vi "HW 2-2_old.vi"() -> ()   [LabVIEW 2017]
panel:
  in  "MR":bool
  in  "+/-":bool
  out "計算機執行時間":string caption="Elapsed Time Text"
  in  "CE":bool
  in  "1/x":bool
  in  "stop":bool
  out "系統時間":timestamp
  in  ".":bool
  out "String":string
  in  "/":bool
  in  "*":bool
  in  "—":bool
  in  "+":bool
  in  "=":bool
  in  "C":bool
  in  "0":bool
  in  "3":bool
  in  "2":bool
  in  "1":bool
  in  "6":bool
  in  "5":bool
  in  "4":bool
  in  "9":bool
  in  "8":bool
  in  "7":bool
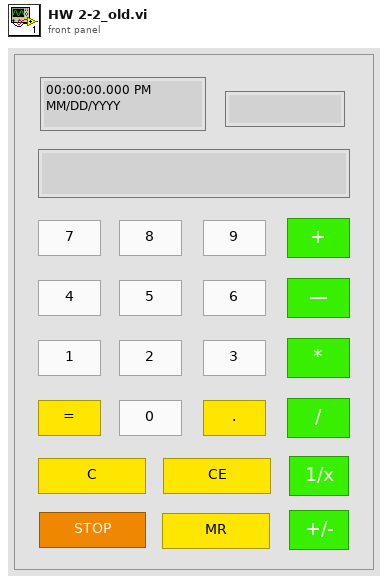
[diagram p1: front panel]
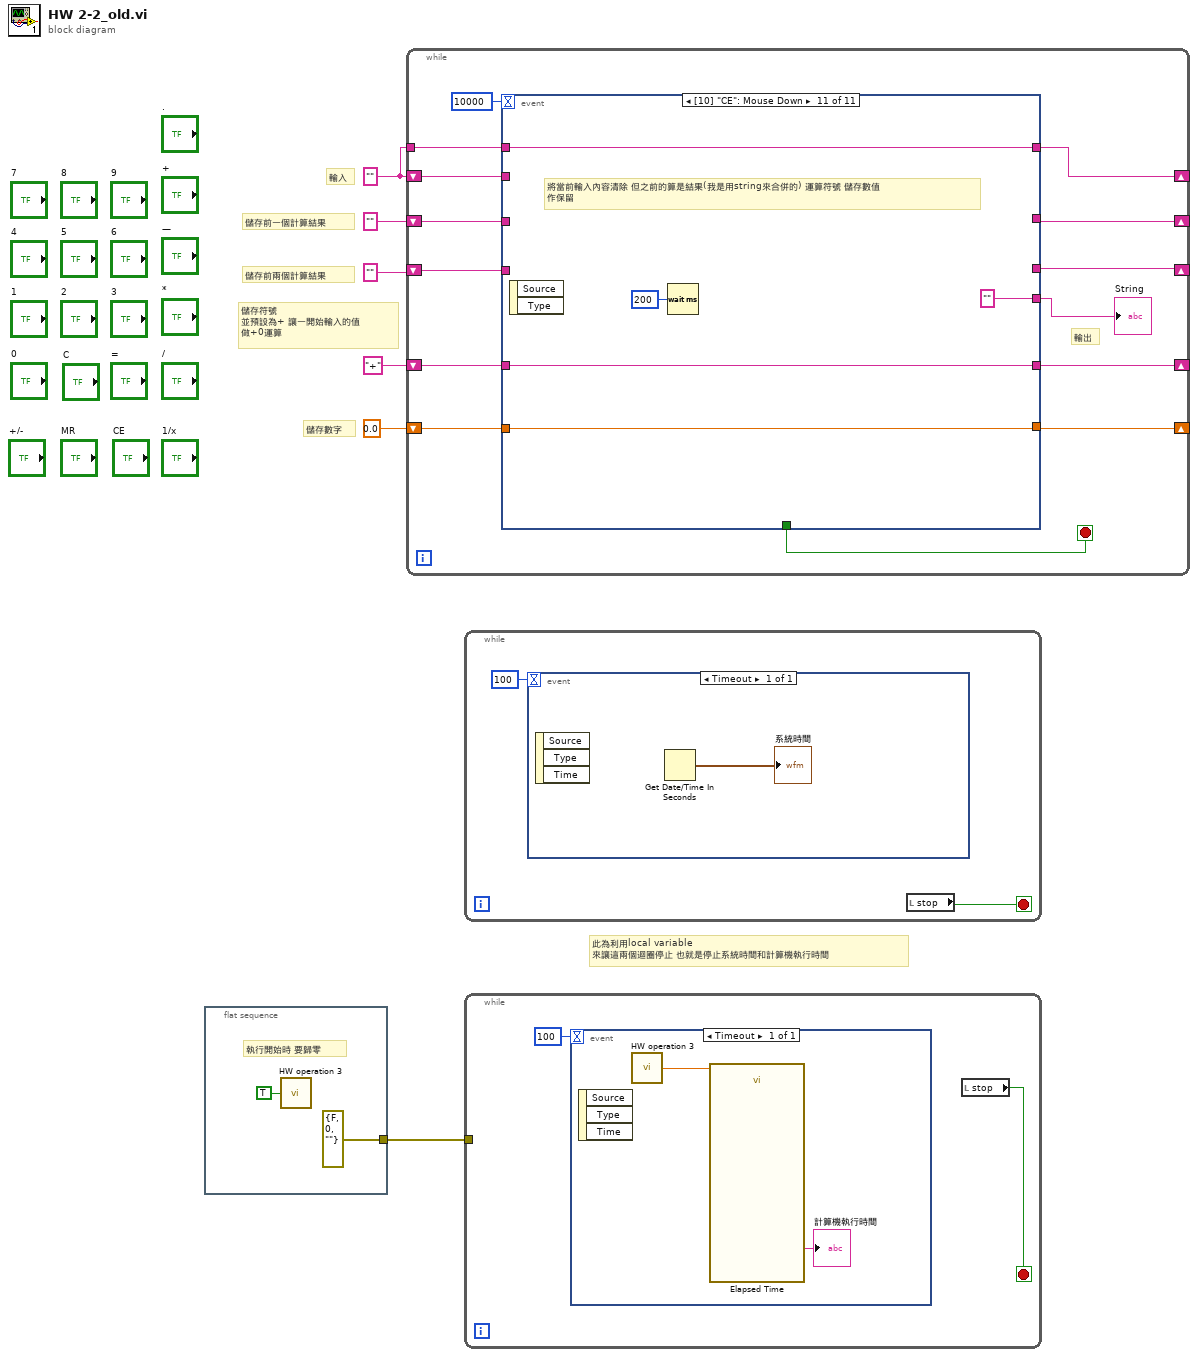
[diagram p0: block diagram]
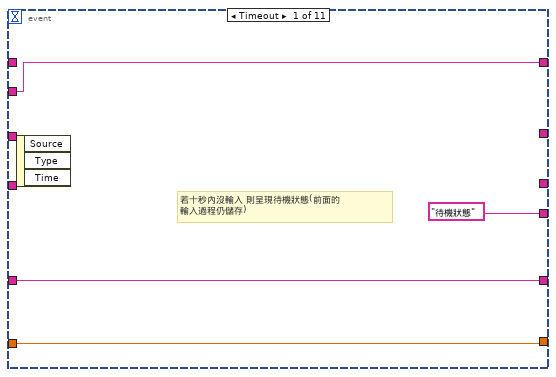
[diagram p2: hidden frame]
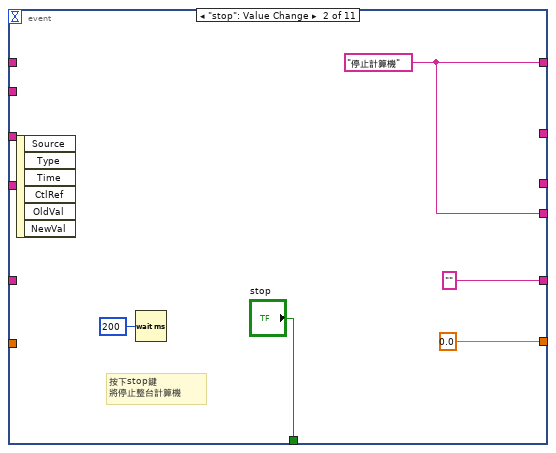
[diagram p3: hidden frame]
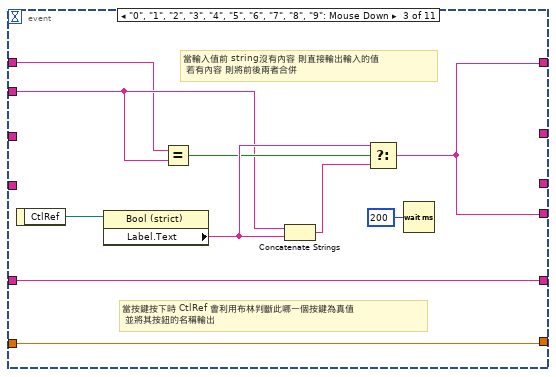
[diagram p4: hidden frame]
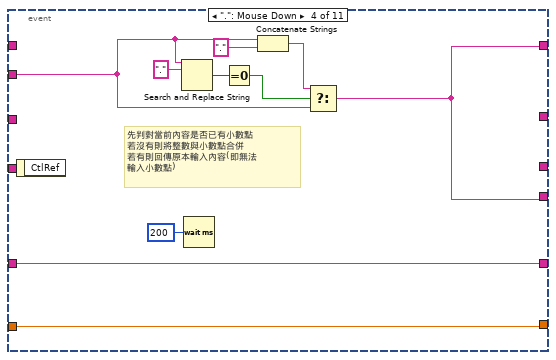
[diagram p5: hidden frame]
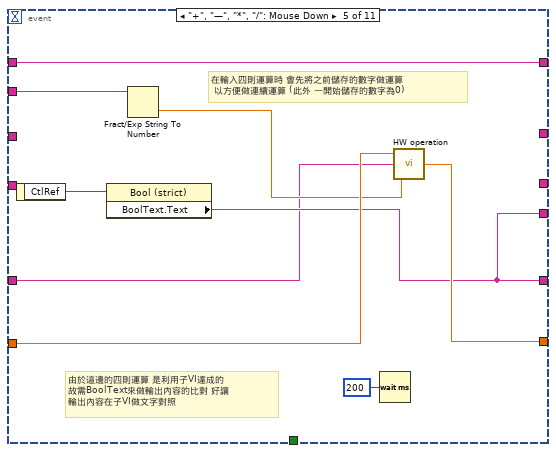
[diagram p6: hidden frame]
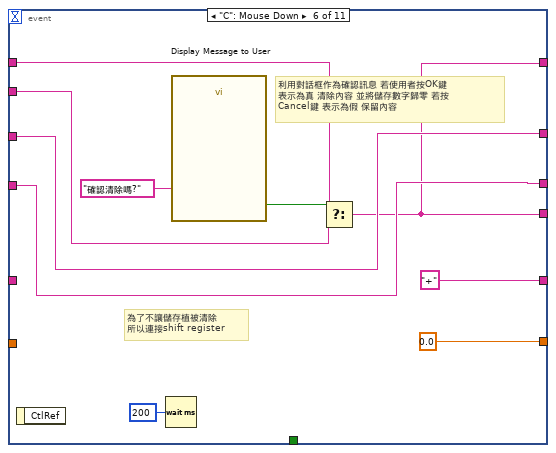
[diagram p7: hidden frame]
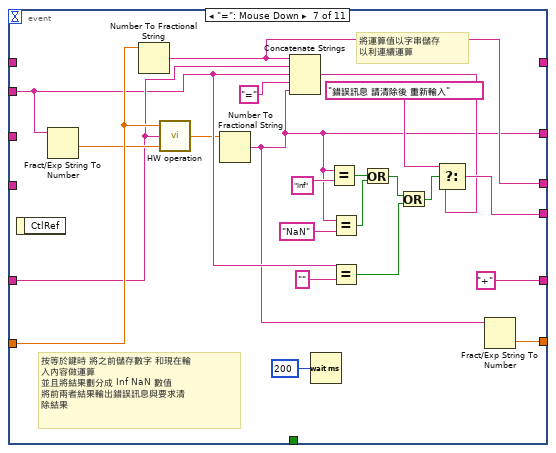
[diagram p8: hidden frame]
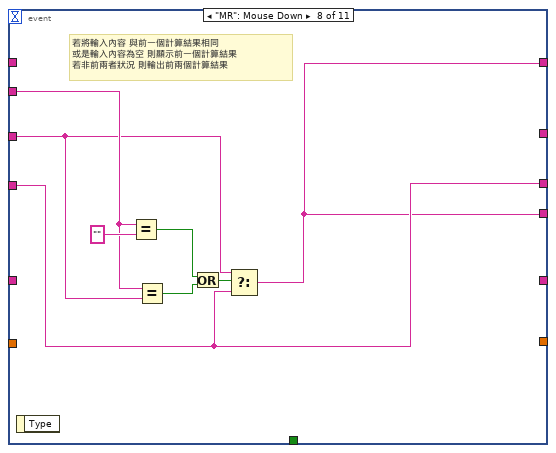
[diagram p9: hidden frame]
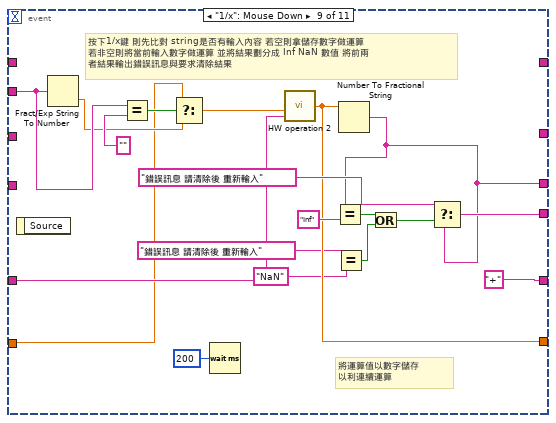
[diagram p10: hidden frame]
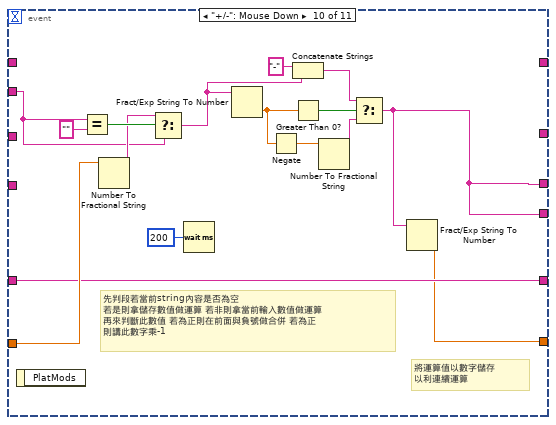
[diagram p11: hidden frame]
diagram:
  w6 = ""
  # "此為利用local variable \n來讓這兩個迴圈停止 也就是停止系統時間和計算機執行時間"
  # "儲存數字"
  # "儲存符號\n並預設為+ 讓一開始輸入的值\n做+0運算"
  # "儲存前兩個計算結果"
  # "儲存前一個計算結果"
  # "輸入"
  n1 = flat-sequence {
    tunnel: [errorcluster {"status"=FALSE, "code"=0, "source"=""} ("error constant")] -> w3
    frame #0 {
      # "執行開始時 要歸零"
      n2 = call "HW operation 3.vi"("stop"=TRUE) -> ()  [unwired: 1 out]
    }
  }
  n3 = while {
    shift-right: [w17] -> _
    shift-left: w6 -> [w15]
    tunnel: w6 -> [w22]
    shift-right: [w18] -> _
    shift-left: "+" -> [w21]
    shift-right: [w19] -> _
    shift-left: 0.0 -> [w20]
    shift-right: [w11] -> _
    shift-left: "" -> [w12]
    shift-right: [w9] -> _
    shift-left: "" -> [w10]
    stop <- w14 stop-if-true
    # "輸出"
    n4 = event shown="[10] \"CE\": Mouse Down" {
      selector: _ -> [_ _ _ _ _ _ _ _ _ _ _]
      dyn-events: _ -> [_ _ _ _ _ _ _ _ _ _ _]
      timeout: 10000 -> [_ _ _ _ _ _ _ _ _ _ _]
      tunnel: w15 -> [w24 _ w37 w43 w55 w65 w78 w97 w116 w122 _]
      tunnel: w22 -> [_ _ w33 _ w58 w66 _ _ _ _ w137]
      tunnel: [w24 w29 w32 w42 w58 w61 _ w98 _ _ w137] -> w17
      tunnel: w21 -> [w26 _ w36 w46 w52 _ w79 _ w114 w123 w139]
      tunnel: w20 -> [w25 _ w35 w45 w57 _ w90 _ w109 w126 w138]
      tunnel: [w25 0.0 ("results") w35 w45 w54 0.0 w73 _ w108 w121 w138] -> w19
      tunnel: [w26 "" ("BoolText.Text") w36 w46 w53 "+" ("BoolText.Text") "+" ("BoolText.Text") _ "+" ("BoolText.Text") w123 w139] -> w18
      tunnel: ["待機狀態" w29 w32 w42 w53 w61 w75 w98 w102 w120 ""] -> w16
      tunnel: [_ "stop" _ _ _ _ _ _ _ _ _] -> w14
      tunnel: w12 -> [_ _ _ _ _ w63 _ w96 _ _ _]
      tunnel: [_ _ _ _ _ w63 w71 _ _ _ _] -> w11
      tunnel: w10 -> [_ _ _ _ _ w62 _ w99 _ _ _]
      tunnel: [_ _ _ _ _ w62 w76 w99 w101 w120 _] -> w9
      event Timeout {
        # "若十秒內沒輸入 則呈現待機狀態(前面的\n輸入過程仍儲存)"
        n5 = event-data() -> ()  [unwired: 1 in, 3 out]
      }
      event "stop": Value Change {
        w29 = "停止計算機" ("Label.Text")
        # "按下stop鍵\n將停止整台計算機"
        n6 = event-data() -> ()  [unwired: 1 in, 6 out]
        n7 = Wait (ms)(milliseconds to wait=u32 200) -> ()  [unwired: 1 out]
      }
      event "0", "1", "2", "3", "4", "5", "6", "7", "8", "9": Mouse Down {
        # "當按鍵按下時 CtlRef 會利用布林判斷此哪一個按鍵為真值\n 並將其按鈕的名稱輸出"
        # "當輸入值前 string沒有內容 則直接輸出輸入的值\n 若有內容 則將前後兩者合併"
        n8 = event-data() -> ("CtlRef"=w41:refnum<vi>)  [unwired: 1 in]
        n9 = property class="Bool (strict)"(reference=w41) -> ("Label.Text"=w40:string)  [unwired: 1 in, 2 out]
        n10 = Equal?(x=w33, y=w37) -> (x = y?=w38:bool)
        n11 = Concatenate Strings(w37, w40) -> (w39:string)
        n12 = Select(t=w40, s=w38, f=w39) -> (s? t:f=w32:string)
        n13 = Wait (ms)(milliseconds to wait=u32 200) -> ()  [unwired: 1 out]
      }
      event ".": Mouse Down {
        # "先判對當前內容是否已有小數點\n若沒有則將整數與小數點合併 \n若有則回傳原本輸入內容(即無法\n輸入小數點)"
        n14 = event-data() -> ()  [unwired: 1 in, 1 out]
        n15 = Search and Replace String(input string=w43, search string=".") -> (number of replacements=w50:i32)  [unwired: 6 in, 3 out]
        n16 = Wait (ms)(milliseconds to wait=u32 200) -> ()  [unwired: 1 out]
        n17 = Equal To 0?(x=w50) -> (x = 0?=w49:bool)
        n18 = Concatenate Strings(w43, "." ("search string")) -> (w48:string)
        n19 = Select(t=w48, s=w49, f=w43) -> (s? t:f=w42:string)
      }
      event "+", "—", "*", "/": Mouse Down {
        # "由於這邊的四則運算 是利用子VI達成的 \n故需BoolText來做輸出內容的比對 好讓\n輸出內容在子VI做文字對照"
        # "在輸入四則運算時 會先將之前儲存的數字做運算\n 以方便做連續運算 (此外 一開始儲存的數字為0)"
        n20 = event-data() -> ("CtlRef"=w60:refnum<vi>)  [unwired: 1 in]
        n21 = property class="Bool (strict)"(reference=w60) -> ("BoolText.Text"=w53:string)  [unwired: 1 in, 2 out]
        n22 = Fract/Exp String To Number(string=w55) -> (number=w56:dbl)  [unwired: 3 in, 1 out]
        n23 = Wait (ms)(milliseconds to wait=u32 200) -> ()  [unwired: 1 out]
        n24 = call "HW operation.vi"("operation2"=w56, "operation"=w52, "operation1"=w57) -> ("results"=w54:dbl)
      }
      event "C": Mouse Down {
        # "為了不讓儲存植被清除\n所以連接shift register"
        # "利用對話框作為確認訊息 若使用者按OK鍵\n表示為真 清除內容 並將儲存數字歸零 若按\nCancel鍵 表示為假 保留內容"
        n25 = event-data() -> ()  [unwired: 1 in, 1 out]
        n26 = Wait (ms)(milliseconds to wait=u32 200) -> ()  [unwired: 1 out]
        n27 = call "Display Message to User"("Message"="確認清除嗎?") -> ("OK"=w67:bool)  [unwired: 9 in, 1 out]
        n28 = Select(t=w66, s=w67, f=w65) -> (s? t:f=w61:string)
      }
      event "=": Mouse Down {
        # "將運算值以字串儲存\n以利連續運算"
        # "按等於鍵時 將之前儲存數字 和現在輸\n入內容做運算\n並且將結果劃分成 Inf NaN 數值\n將前兩者結果輸出錯誤訊息與要求清\n除結果"
        n29 = event-data() -> ()  [unwired: 1 in, 1 out]
        n30 = Fract/Exp String To Number(string=w78) -> (number=w89:dbl)  [unwired: 3 in, 1 out]
        n31 = Number To Fractional String(number=w90) -> (F-format string=w76:string)  [unwired: 3 in]
        n32 = call "HW operation.vi"("operation2"=w89, "operation"=w79, "operation1"=w90) -> ("results"=w74:dbl)
        n33 = Number To Fractional String(number=w74) -> (F-format string=w71:string)  [unwired: 3 in]
        n34 = Concatenate Strings(w76, w79, w78, "=", w71) -> (w72:string)
        n35 = Wait (ms)(milliseconds to wait=u32 200) -> ()  [unwired: 1 out]
        n36 = Equal?(x=w71, y="Inf") -> (x = y?=w85:bool)
        n37 = Equal?(x=w71, y="NaN") -> (x = y?=w84:bool)
        n38 = Equal?(x=w78, y="") -> (x = y?=w81:bool)
        n39 = Or(x=w85, y=w84) -> (x .or. y?=w82:bool)
        n40 = Or(x=w82, y=w81) -> (x .or. y?=w80:bool)
        n41 = Select(t="錯誤訊息 請清除後 重新輸入", s=w80, f=w72) -> (s? t:f=w75:string)
        n42 = Fract/Exp String To Number(string=w71) -> (number=w73:dbl)  [unwired: 3 in, 1 out]
      }
      event "MR": Mouse Down {
        # "若將輸入內容 與前一個計算結果相同\n或是輸入內容為空 則顯示前一個計算結果\n若非前兩者狀況 則輸出前兩個計算結果"
        n43 = event-data() -> ()  [unwired: 1 in, 1 out]
        n44 = Equal?(x=w97, y="") -> (x = y?=w94:bool)
        n45 = Equal?(x=w97, y=w96) -> (x = y?=w93:bool)
        n46 = Or(x=w94, y=w93) -> (x .or. y?=w95:bool)
        n47 = Select(t=w96, s=w95, f=w99) -> (s? t:f=w98:string)
      }
      event "1/x": Mouse Down {
        # "將運算值以數字儲存 以利連續運算"
        # "按下1/x鍵 則先比對 string是否有輸入內容 若空則拿儲存數字做運算\n若非空則將當前輸入數字做運算 並將結果劃分成 Inf NaN 數值 將前兩\n者結果輸出錯誤訊息與要求清除結果"
        n48 = event-data() -> ()  [unwired: 1 in, 1 out]
        n49 = Fract/Exp String To Number(string=w116) -> (number=w115:dbl)  [unwired: 3 in, 1 out]
        n50 = Equal?(x=w116, y="") -> (x = y?=w118:bool)
        n51 = Select(t=w109, s=w118, f=w115) -> (s? t:f=w113:dbl)
        n52 = Wait (ms)(milliseconds to wait=u32 200) -> ()  [unwired: 1 out]
        n53 = call "HW operation 2.vi"("Combo Box"=w114, "Numeric"=w113) -> ("Numeric 2"=w108:dbl)  [unwired: 1 out]
        n54 = Equal?(x="錯誤訊息 請清除後 重新輸入", y="NaN") -> (x = y?=w103:bool)
        n55 = Number To Fractional String(number=w108) -> (F-format string=w101:string)  [unwired: 3 in]
        n56 = Equal?(x=w101, y="Inf") -> (x = y?=w105:bool)
        n57 = Or(x=w105, y=w103) -> (x .or. y?=w104:bool)
        n58 = Select(t="錯誤訊息 請清除後 重新輸入", s=w104, f=w101) -> (s? t:f=w102:string)
      }
      event "+/-": Mouse Down {
        # "將運算值以數字儲存 以利連續運算"
        # "先判段若當前string內容是否為空\n若是則拿儲存數值做運算 若非則拿當前輸入數值做運算\n再來判斷此數值 若為正則在前面與負號做合併 若為正 \n則講此數字乘-1"
        n59 = event-data() -> ()  [unwired: 1 in, 1 out]
        n60 = Equal?(x=w122, y="") -> (x = y?=w127:bool)
        n61 = Number To Fractional String(number=w126) -> (F-format string=w124:string)  [unwired: 3 in]
        n62 = Select(t=w124, s=w127, f=w122) -> (s? t:f=w125:string)
        n63 = Wait (ms)(milliseconds to wait=u32 200) -> ()  [unwired: 1 out]
        n64 = Fract/Exp String To Number(string=w125) -> (number=w133:dbl)  [unwired: 3 in, 1 out]
        n65 = Negate(x=w133) -> (-x=w132:dbl)
        n66 = Concatenate Strings("-" ("string"), w125) -> (w131:string)
        n67 = Greater Than 0?(x=w133) -> (x > 0?=w135:bool)
        n68 = Number To Fractional String(number=w132) -> (F-format string=w130:string)  [unwired: 3 in]
        n69 = Select(t=w131, s=w135, f=w130) -> (s? t:f=w120:string)
        n70 = Fract/Exp String To Number(string=w120) -> (number=w121:dbl)  [unwired: 3 in, 1 out]
      }
      event "CE": Mouse Down {
        # "將當前輸入內容清除 但之前的算是結果(我是用string來合併的) 運算符號 儲存數值\n作保留"
        n71 = event-data() -> ()  [unwired: 1 in, 2 out]
        n72 = Wait (ms)(milliseconds to wait=u32 200) -> ()  [unwired: 1 out]
      }
    }
    "String" <- w16
  }
  n73 = while {
    stop <- w141 stop-if-true
    n74 = event shown="[0] Timeout" {
      selector: _ -> [_]
      dyn-events: _ -> [_]
      timeout: 100 -> [_]
      event Timeout {
        n75 = event-data() -> ()  [unwired: 1 in, 3 out]
        n76 = Get Date/Time In Seconds() -> (seconds since 1Jan1904=→"系統時間":timestamp)
      }
    }
    n77 = local read "stop"() -> (w141:bool)
  }
  n78 = while {
    tunnel: w3 -> [_]
    stop <- w145 stop-if-true
    n79 = event shown="[0] Timeout" {
      selector: _ -> [_]
      dyn-events: _ -> [_]
      timeout: 100 -> [_]
      event Timeout {
        n80 = event-data() -> ()  [unwired: 1 in, 3 out]
        n81 = call "HW operation 3.vi"() -> ("Numeric"=w146:dbl)  [unwired: 1 in]
        n82 = call "Elapsed Time"("Time Target (s)"=w146) -> ("Elapsed Time Text"=→"計算機執行時間":string)  [unwired: 11 in, 7 out]
      }
    }
    n83 = local read "stop"() -> (w145:bool)
  }
